vi "Poll for Reset Monitor.vi"(0 "GEA2 Reference In":refnum<k24>, 7 "Status":enum16{"Clear", "Set"}(ring), 11 "Error In":errorcluster) -> (4 "GEA2 Reference Out":refnum<k24>, 6 "Pass/Fail?":bool, 8 "Report Text":string, 10 "Time until condition met (s)":dbl, 15 "Error Out":errorcluster)   [LabVIEW 2018]
uses:
  D:/Common/LabVIEW GEA2 Toolkit/source/GEA3 DLL Source/GeaCommunication.dll
  Common/LabVIEW GEA2 Toolkit/source/GEA3 DLL Source/GeaCommunication.dll
  Common/LabVIEW GEA2 Toolkit/GEA3/type defs/Source_Destination.ctl
  Common/LabVIEW GEA2 Toolkit/GEA3/type defs/ERD Read Data In.ctl
  Common/LabVIEW GEA2 Toolkit/GEA3/type defs/Data Type.ctl
  C:/Users/iallatyp/Desktop/New folder/GEA3/library/GEA2_Toolkit.lvlib
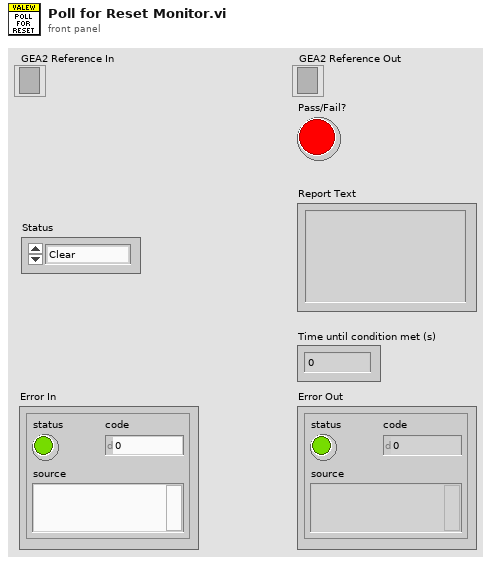
[diagram p1: front panel]
types:
  T1 = typedef "GEA2_Toolkit.lvlib/Source_Destination.ctl" = cluster{"Source":u8, "Destination":u8}
  T2 = typedef "GEA2_Toolkit.lvlib/ERD Read Data In.ctl" = cluster{"ERD Number":u16, "Data Type":T3}
  T3 = typedef "GEA2_Toolkit.lvlib/Data Type.ctl" = enum16{"string", "boolean", "uint8_t", "uint16_t", "uint32_t", "uint64_t", "int8_t", "int16_t", "int32_t", "int64_t"}
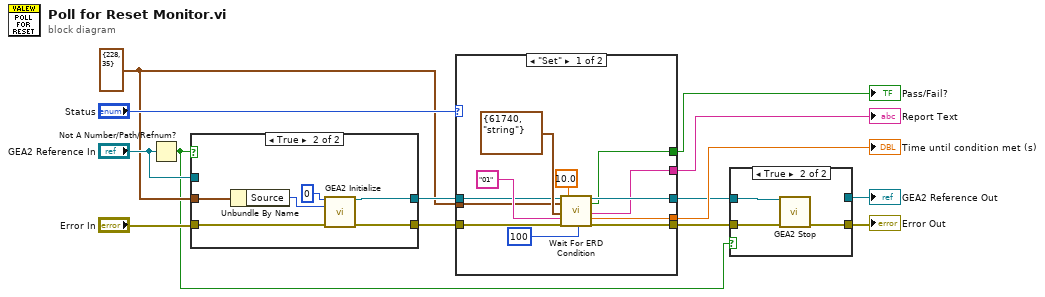
[diagram p0: block diagram]
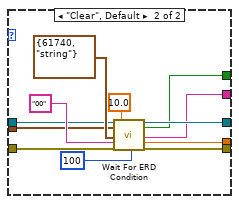
[diagram p2: hidden frame]
diagram:
  w8 = T1 {"Source"=228, "Destination"=35} ("GEA Inputs")
  n1 = Not A Number/Path/Refnum?(number/path/refnum="GEA2 Reference In") -> (NaN/Path/Refnum?=w5:bool)
  n2 = case shown="True" w5 {
    tunnel: "Error In" -> [w16 w22]
    tunnel: [w16 w21] -> w12
    tunnel: [w15 w20] -> w9
    tunnel: w8 -> [_ w18]
    tunnel: "GEA2 Reference In" -> [w15 _]
    frame False {
    }
    frame True {
      n3 = Unbundle By Name(w18) -> ("Source"=w19:u8)
      n4 = call "GEA2 Initialize.vi"("Board Index"=0, "Source Address"=w19, "error in"=w22) -> ("GEA2 Reference Out"=w20:refnum<k24>, "error out"=w21:errorcluster)  [unwired: 10 in, 1 out]
    }
  }
  n5 = case shown="\"Set\"" "Status" {
    tunnel: [w31 w43] -> w14
    tunnel: w12 -> [w30 w42]
    tunnel: w8 -> [w28 w40]
    tunnel: w9 -> [w27 w39]
    tunnel: [w26 w38] -> w7
    tunnel: [w24 w37] -> w1
    tunnel: [w23 w36] -> w2
    tunnel: [w25 w35] -> w6
    frame "Set" {
      n6 = call "Wait For ERD Condition.vi"("GEA2 Reference In"=w27, "GEA Inputs"=w28, "ERD Read Data"=T2 {"ERD Number"=61740, "Data Type"=enum."string"}, "Expected Low"="01", "Error In"=w30, "Timeout (s)"=10.0, "Loop Rate (ms)"=u32 100) -> ("GEA2 Reference Out"=w26:refnum<k24>, "Pass/Fail?"=w24:bool, "Report Text"=w23:string, "Execution Time"=w31:dbl, "Error Out"=w25:errorcluster)  [unwired: 8 in]
    }
    frame "Clear", Default {
      n7 = call "Wait For ERD Condition.vi"("GEA2 Reference In"=w39, "GEA Inputs"=w40, "ERD Read Data"=T2 {"ERD Number"=61740, "Data Type"=enum."string"}, "Expected Low"="00", "Error In"=w42, "Timeout (s)"=10.0, "Loop Rate (ms)"=u32 100) -> ("GEA2 Reference Out"=w38:refnum<k24>, "Pass/Fail?"=w37:bool, "Report Text"=w36:string, "Execution Time"=w43:dbl, "Error Out"=w35:errorcluster)  [unwired: 8 in]
    }
  }
  "Time until condition met (s)" <- w14
  "Pass/Fail?" <- w1
  "Report Text" <- w2
  n8 = case shown="True" w5 {
    tunnel: [w47 w51] -> w4
    tunnel: w7 -> [w48 w50]
    tunnel: w6 -> [w47 w49]
    tunnel: [w48 _] -> w3
    frame False {
    }
    frame True {
      n9 = call "GEA2 Stop.vi"("GEA2 Reference In"=w50, "Error In"=w49) -> ("Error Out"=w51:errorcluster)  [unwired: 13 in]
    }
  }
  "GEA2 Reference Out" <- w3
  "Error Out" <- w4
